vi "Set Gain [GAN].vi"(7 "Micropulse # In":i32, 8 "error in (no error)":errorcluster, 9 "Gain (dB)":dbl caption="[GAN]" min=-6.0 max=70.0 step=0.25 format="%.2fdB", 11 "Test Number":u32) -> (0 "error out":errorcluster, 5 "Micropulse # Out":i32)   [LabVIEW 2026, in "MicroPulse_Driver.lvlib"]
doc: "Sets the absolute gain for the test number specified\n\nParameters:\n<Tn> : Test number. An integer value from 0 to the maximum number of tests (default maximum is 1279 tests).\nTn = 0 for all conventional tests. If the S extension is used it applies to all tests in the sweep number specified: 1-32, 0 = all sweeps.\n\n<Value> : Integer in the range 0 to 280, each increment corresponding to 0.25dB.\n\nExample: GAN 0 80 : Adjusts gain for all tests within the set NUM to 20dB."
uses:
  MicroPulse_Driver.lvlib
  Private/MP-Registry Action-Enum.ctl
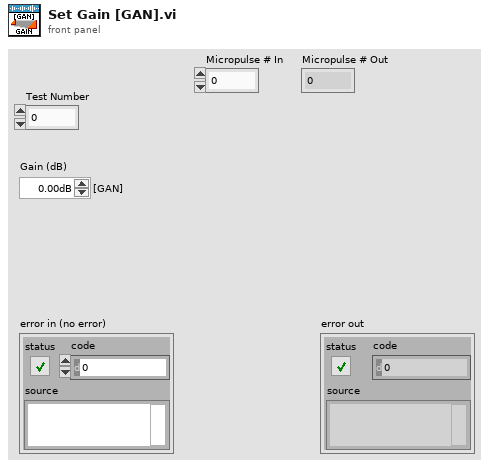
[diagram p1: front panel]
types:
  T1 = typedef "MicroPulse_Driver.lvlib/MP-Registry Action-Enum.ctl" = enum16{"Read", "Add Test", "Add Command", "Add Gate Command", "Add Encoder Command", "Clear Command  List", "Set Registry", "Set System Details", "Set DOF", "Set Velocity", "Disable Asynch Reads", "Enable Asynch Reads", "Add Connection", "Disconnect", "Shutdown"}
  T2 = typedef "MicroPulse_Driver.lvlib/TCP config.ctl" = cluster{"Connection ID":refnum<k5>, "IP address":string, "host port":u16, "OC timeout":i32, "Read timeout":i32, "Write timeout":i32}
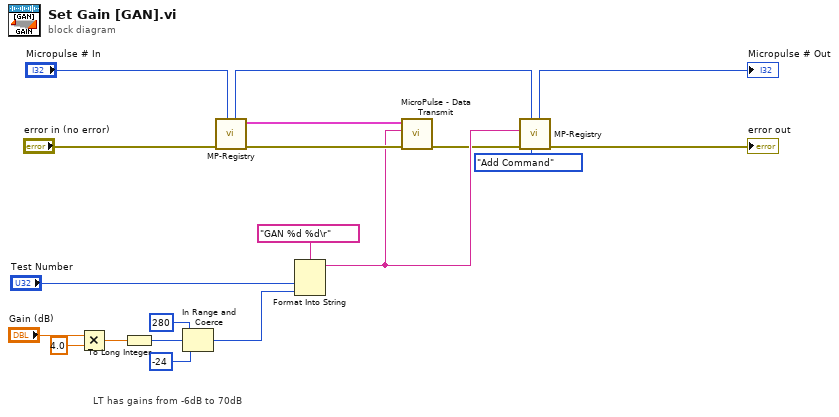
[diagram p0: block diagram]
diagram:
  # "LT has gains from -6dB to 70dB"
  n1 = Multiply(x="Gain (dB)", y=4.0) -> (x*y=w3:dbl)
  n2 = To Long Integer(number=w3) -> (32bit integer=w1:i32)
  n3 = In Range and Coerce(upper limit=280, x=w1, lower limit=-24) -> (coerced(x)=w6:i32)  [unwired: 1 out]
  n4 = call "MP-Registry.vi"("Micropulse # In"="Micropulse # In", "error in (no error)"="error in (no error)") -> ("error out"=w17:errorcluster, "TCP config"=w16:T2, "Micropulse # Out"=w9:i32)  [unwired: 6 in, 1 out]
  n5 = Format Into String(format string="GAN %d %d\r", "Test Number", w6) -> (resulting string=w13:string)  [unwired: 2 in, 1 out]
  n6 = call "MicroPulse - Data Transmit.vi"("error in (no error)"=w17, "data"=w13, "TCP config"=w16) -> ("error out"=w11:errorcluster)  [unwired: 6 in, 2 out]
  n7 = call "MP-Registry.vi"("Action"=MP-Registry_Action-Enum."Add Command", "Micropulse # In"=w9, "error in (no error)"=w11, "Data in"=w13) -> ("error out"=→"error out":errorcluster, "Micropulse # Out"=→"Micropulse # Out":i32)  [unwired: 4 in, 2 out]
